vi "Read CSPP_DataCollection out.vi"(8 "error in (no error)":errorcluster, 11 "Readout Msg in":refnum<class "Readout Msg.lvclass">) -> (0 "error out":errorcluster, 2 "CSPP_BaseClasses.lvlib:CSPP_DataCollection.lvclass":refnum<class "CSPP_DataCollection.lvclass">, 3 "Readout Msg out":refnum<class "Readout Msg.lvclass">)   [LabVIEW 2021, in "BNT_ULx.lvlib" / "Readout Msg.lvclass"]
uses:
  Readout Msg.lvclass
  CSPP_Core/Classes/CSPP_BaseClasses/DataCollection/CSPP_DataCollection.lvclass
  Readout Msg.lvclass/Readout Msg.ctl
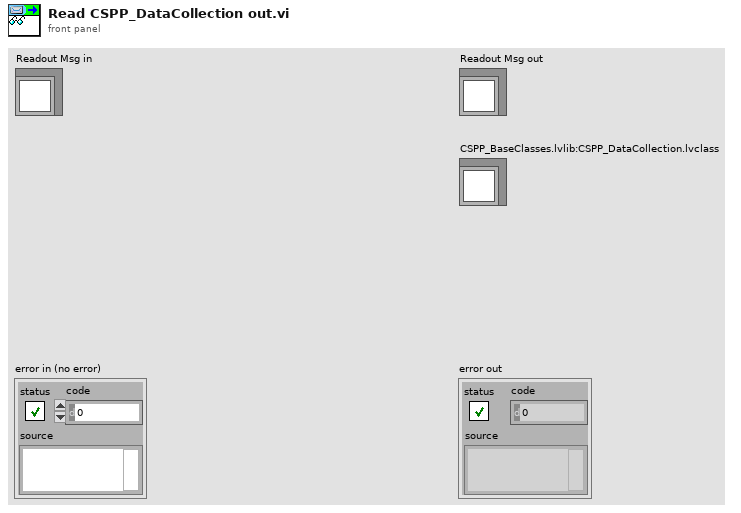
[diagram p1: front panel]
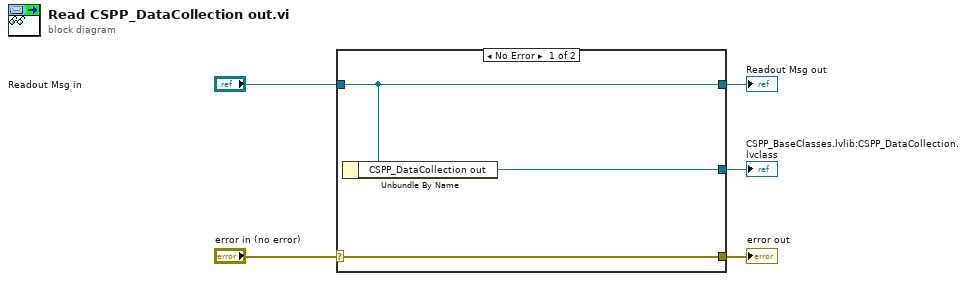
[diagram p0: block diagram]
diagram:
  n1 = case shown="No Error" "error in (no error)" {
    selector: "error in (no error)" -> [w8 w9]
    tunnel: [w8 w9] -> w4
    tunnel: [w7 w10] -> w2
    tunnel: "Readout Msg in" -> [w7 w10]
    tunnel: [w6 _] -> w1
    frame No Error {
      n2 = Unbundle By Name(w7) -> ("CSPP_DataCollection out"=w6:refnum<class "CSPP_DataCollection.lvclass">)
    }
    frame Error {
    }
  }
  "error out" <- w4
  "Readout Msg out" <- w2
  "CSPP_BaseClasses.lvlib:CSPP_DataCollection.lvclass" <- w1
